vi "WriteSensorData.vi"(8 "error in (no error)":errorcluster, 10 "SensorDataInput":variant, 11 "ModuleID":i32) -> (0 "error out":errorcluster)   [LabVIEW 2014, in "AnalysisPlugins.lvlib" / "AnalysisPluginsBase.lvclass"]
uses:
  AnalysisPluginsBase.lvclass
  AnalysisModule/Protected/clEventType.ctl
  <vilib>/Utility/error.llb/Error Cluster From Error Code.vi
  <vilib>/ErrorRing/Error Ring.xnode
  AnalysisModule/AnalysisModule.lvlib
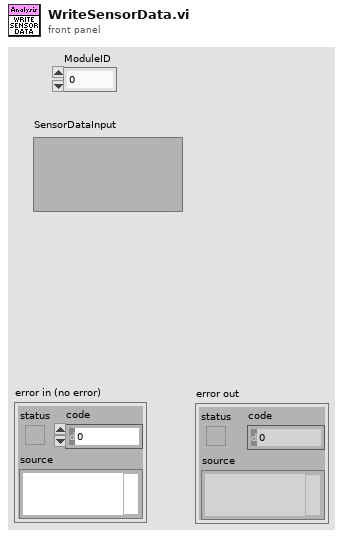
[diagram p1: front panel]
types:
  T1 = typedef "AnalysisModule.lvlib/clRequestEvents.ctl" = cluster{"StopRequest":refnum<user-event>, "PathToINI":refnum<user-event>, " LoadPlugin":refnum<user-event>, "ShowPanel":refnum<user-event>, "WriteSamples":refnum<user-event>, "ReadConfig":refnum<user-event>, "WriteConfig":refnum<user-event>, "WriteSignalParams":refnum<user-event>, "WriteTestType":refnum<user-event>, "WriteFileName":refnum<user-event>, "WriteMagCorr":refnum<user-event>, "WriteDlyCorr":refnum<user-event>, "ConfigDlg":refnum<user-event>, "WriteSensorData":refnum<user-event>, "Initialize":refnum<user-event>, "Abort":refnum<user-event>}
  T2 = typedef "AnalysisModule.lvlib/clEventType.ctl" = cluster{"ModuleID":i32, "Data":variant}
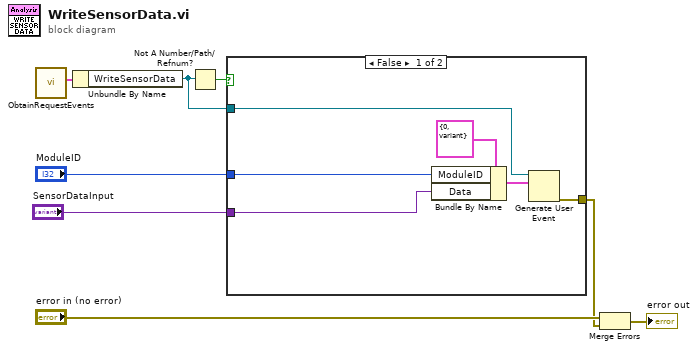
[diagram p0: block diagram]
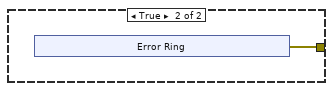
[diagram p2: hidden frame]
diagram:
  n1 = call "ObtainRequestEvents.vi"() -> ("AnalysisRequestEvents"=w8:T1)  [unwired: 10 in, 1 out]
  n2 = Unbundle By Name(w8) -> ("WriteSensorData"=w5:refnum<user-event>)
  n3 = Not A Number/Path/Refnum?(number/path/refnum=w5) -> (NaN/Path/Refnum?=w6:bool)
  n4 = case shown="False" w6 {
    tunnel: "SensorDataInput" -> [w9 _]
    tunnel: w5 -> [w11 _]
    tunnel: "ModuleID" -> [w13 _]
    tunnel: [w10 w15] -> w1
    frame False {
      n5 = Bundle By Name(cluster=T2 {"ModuleID"=0, "Data"=variant} ("clEventType"), "ModuleID"=w13, "Data"=w9) -> (w12:T2)
      n6 = Generate User Event(user event=w11, event data cluster=w12) -> (error out=w10:errorcluster)  [unwired: 2 in, 1 out]
    }
    frame True {
      n7 = xnode "Error Ring"() -> ("error out"=w15:errorcluster)
    }
  }
  n8 = Merge Errors("error in (no error)", w1) -> (→"error out":errorcluster)
